vi "Set Blueprint Qty.vi"(8 "error in (no error)":errorcluster, 9 "Qty":dbl, 10 "Blueprint":refnum<class "Blueprint.lvclass">, 11 "App in":refnum<class "App.lvclass">) -> (0 "error out":errorcluster, 3 "App out":refnum<class "App.lvclass">)   [LabVIEW 2020, in "App.lvclass"]
uses:
  App.lvclass
  Blueprint/Blueprint.lvclass
  App.lvclass/App.ctl
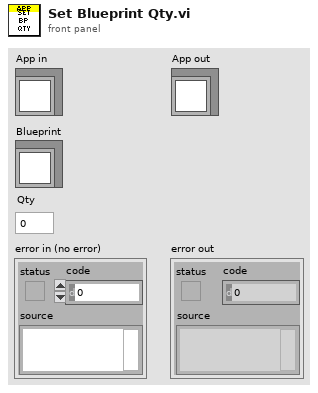
[diagram p1: front panel]
types:
  T1 = typedef "App.lvclass/Blueprint Qty.ctl" = cluster{"Blueprint":refnum<class "Blueprint.lvclass">, "Qty":dbl}
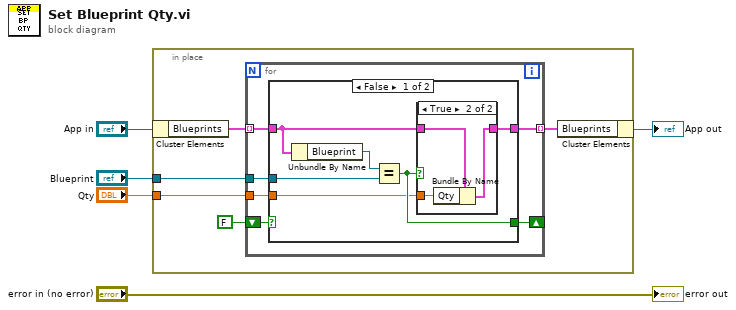
[diagram p0: block diagram]
diagram:
  n1 = in-place {
    in-place-border: "Blueprint" -> [w9]
    in-place-border: "Qty" -> [w8]
    n2 = in-place-cluster #1("App in") -> ("Blueprints"=w10:T1[])
    n3 = for {
      tunnel: w10 -> [w16] mode=indexing
      tunnel: w9 -> [w15]
      tunnel: w8 -> [w11]
      shift-right: [w13] -> _
      shift-left: FALSE -> [w14]
      tunnel: [w12] -> w6 mode=indexing
      n4 = case shown="False" w14 {
        selector: w14 -> [_ w28]
        tunnel: w16 -> [w19 w27]
        tunnel: w15 -> [w21 _]
        tunnel: [w20 w28] -> w13
        tunnel: [w17 w27] -> w12
        tunnel: w11 -> [w18 _]
        frame False {
          n5 = Unbundle By Name(w19) -> ("Blueprint"=w22:refnum<class "Blueprint.lvclass">)
          n6 = Equal?(x=w22, y=w21) -> (x = y?=w20:bool)
          n7 = case shown="True" w20 {
            tunnel: w19 -> [w23 w26]
            tunnel: w18 -> [_ w25]
            tunnel: [w23 w24] -> w17
            frame False {
            }
            frame True {
              n8 = Bundle By Name(cluster=w26, "Qty"=w25) -> (w24:T1)
            }
          }
        }
        frame True {
        }
      }
    }
    n9 = in-place-cluster #1("Blueprints"=w6) -> (→"App out":refnum<class "App.lvclass">)
  }
  "error out" <- "error in (no error)"
